vi "_CSMObj-Message Check.vi"(6 "CSM":string, 8 "Error in":errorcluster caption="Error in (no error)", 10 "message":string, 11 "CSMQ in":T1={"Requested Name"="", "Module Name"="", "Mode"=enum."Stand Alone", "Queue"=refnum, "CSM-Data"=refnum, "User Event"=refnum, "Status Change Event"=refnum, "Allowed Messages"=[], "Mode-Data"=refnum, "Group Name"="", "Exit Event"=refnum}) -> (0 "Error out":errorcluster, 2 "message(dup)":string, 3 "CSMQ out":T1={"Requested Name"="", "Module Name"="", "Mode"=enum."Stand Alone", "Queue"=refnum, "CSM-Data"=refnum, "User Event"=refnum, "Status Change Event"=refnum, "Allowed Messages"=[], "Mode-Data"=refnum, "Group Name"="", "Exit Event"=refnum})   [LabVIEW 2020, in "Communicable State Machine.lvlib"]
uses:
  Communicable State Machine.lvlib
  _CSMObj.ctl
  Priority Queue.lvclass
  _CSM_MODE.ctl
  _CSMObj-Data.ctl
  _CSM Status Change Event Data.ctl
  _CSMObj-ModeData.ctl
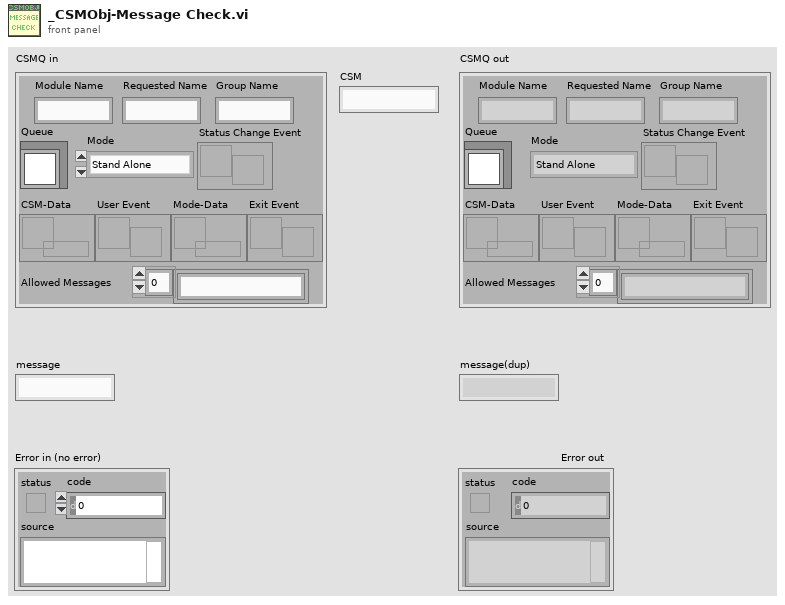
[diagram p1: front panel]
types:
  T1 = typedef "Communicable State Machine.lvlib/_CSMObj.ctl" = cluster{"Requested Name":string, "Module Name":string, "Mode":T2, "Queue":refnum<class "Priority Queue.lvclass">, "CSM-Data":refnum<data-value>, "User Event":refnum<user-event>, "Status Change Event":refnum<user-event>, "Allowed Messages":string[], "Mode-Data":refnum<data-value>, "Group Name":string, "Exit Event":refnum<user-event>}
  T2 = typedef "Communicable State Machine.lvlib/_CSM_MODE.ctl" = enum16{"Not Exist", "Stand Alone", "CSM", "Worker Agent", "Worker", "Chain", "Chain Node"}
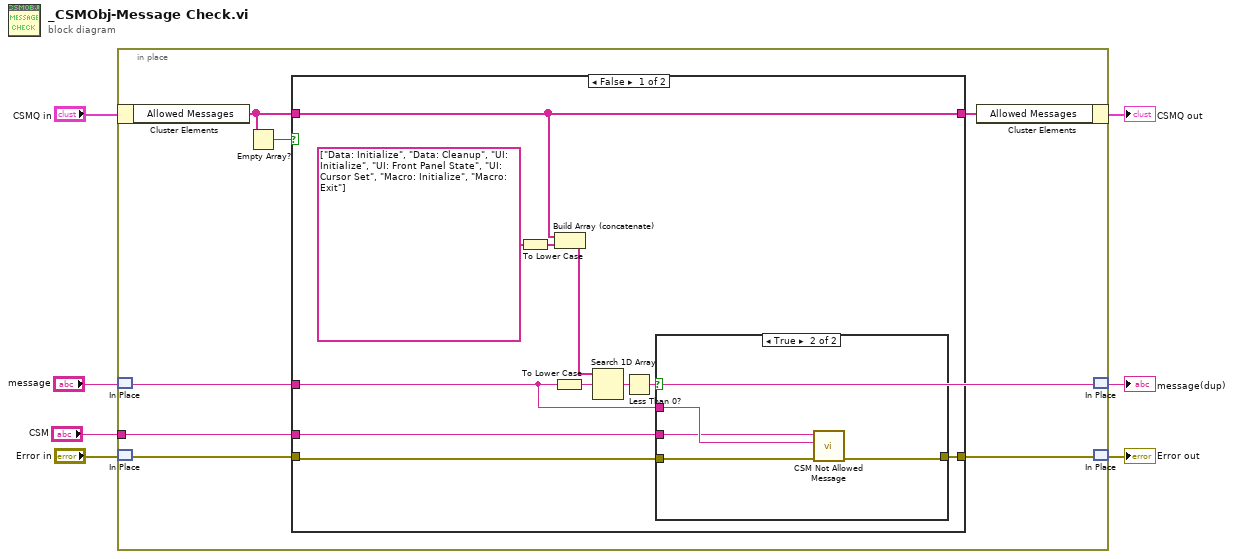
[diagram p0: block diagram]
diagram:
  n1 = in-place "In Place Element Structure" {
    in-place-border: "CSM" -> [w8]
    n2 = in-place-cluster #1("CSMQ in") -> ("Allowed Messages"=w13:string[])
    n3 = in-place-match #2("message") -> (w14:string)
    n4 = in-place-match #3("Error in") -> (w9:errorcluster)
    n5 = Empty Array?(array=w13) -> (empty?=w12:bool)
    n6 = case shown="False" w12 {
      tunnel: w14 -> [w24 _]
      tunnel: w13 -> [w18 w32]
      tunnel: [w18 w32] -> w11
      tunnel: [w22 w31] -> w10
      tunnel: w9 -> [w21 w31]
      tunnel: w8 -> [w15 _]
      frame False {
        n7 = To Lower Case(string=string[] ["Data: Initialize", "Data: Cleanup", "UI: Initialize", "UI: Front Panel State", "UI: Cursor Set", "Macro: Initialize", "Macro: Exit"] ("array")) -> (all lower case string=w17:string[])
        n8 = To Lower Case(string=w24) -> (all lower case string=w20:string)
        n9 = Build Array (concatenate)(w18, w17) -> (w16:string[])
        n10 = Search 1D Array(1D array=w16, element=w20) -> (index of element=w25:i32)  [unwired: 1 in]
        n11 = Less Than 0?(x=w25) -> (x < 0?=w23:bool)
        n12 = case shown="True" w23 {
          tunnel: w24 -> [_ w29]
          tunnel: [w26 w28] -> w22
          tunnel: w21 -> [w26 w30]
          tunnel: w15 -> [_ w27]
          frame False {
          }
          frame True {
            n13 = call "CSM Not Allowed Message.vi"("error in (no error)"=w30, "State"=w29, "CSM"=w27) -> ("error out"=w28:errorcluster)  [unwired: 8 in]
          }
        }
      }
      frame True {
      }
    }
    n14 = in-place-cluster #1("Allowed Messages"=w11) -> (→"CSMQ out":T1)
    n15 = in-place-match #2(w14) -> (→"message(dup)":string)
    n16 = in-place-match #3(w10) -> (→"Error out":errorcluster)
  }
